vi "svx_Matched Index.vi"(11 "channel property":T1[](array[typedef]) {"probe angle [deg]" max=360; "direction" items=["CCW", "CW"]}) -> (0 "single index":i32[](array[numeric]), 1 "single list":u32[](array[numeric]), 2 "pair index":cluster{"index 1":i32, "index 2":i32}[](array[cluster]), 3 "new pair list":u32[](array[numeric]), 4 "direction error":bool, 6 "pair error":bool)   [LabVIEW 2017]
uses:
  <vilib>/addons/Sound and Vibration/Order Analysis/Data Presentation/SubVIs/OAT MCM Channel Property.ctl
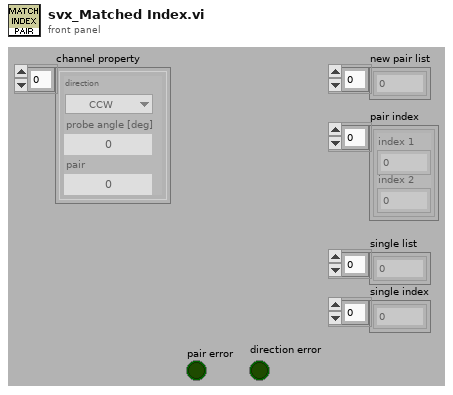
[diagram p1: front panel]
types:
  T1 = typedef "OAT MCM Channel Property.ctl" = cluster{"direction":u16, "probe angle [deg]":u16, "pair":u16}
  T2 = cluster{"index of element":i32, "index of element":i32}[]
  T3 = cluster{"index of element":i32, "index of element":i32}
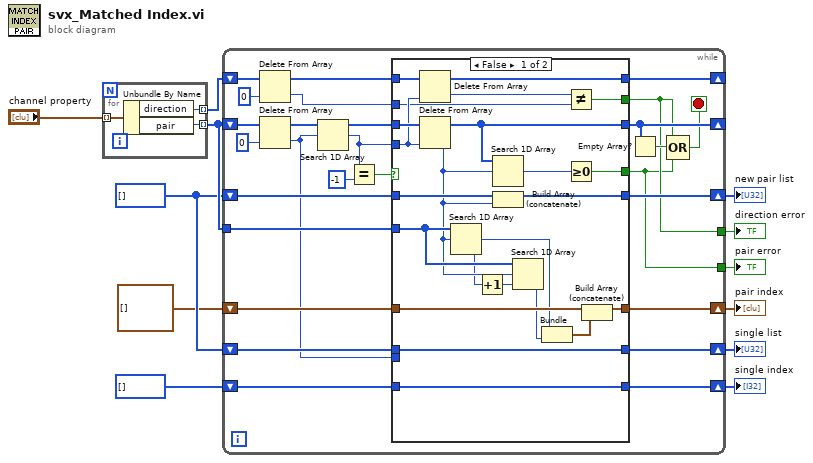
[diagram p0: block diagram]
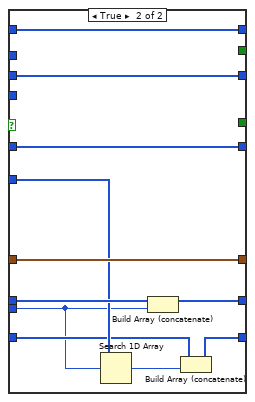
[diagram p2: hidden frame]
diagram:
  w9 = u32[] []
  n1 = for {
    tunnel: "channel property" -> [w15] mode=indexing
    tunnel: [w14] -> w10 mode=indexing
    tunnel: [w13] -> w3 mode=indexing
    n2 = Unbundle By Name(w15) -> ("direction"=w13:u16, "pair"=w14:u16)
  }
  n3 = while {
    shift-right: [w35] -> _
    shift-left: w10 -> [w34]
    shift-right: [w37] -> w11
    shift-left: w9 -> [w36]
    shift-right: [w33] -> w4
    shift-left: T2 [] -> [w32]
    tunnel: w10 -> [w31]
    shift-right: [w29] -> w6
    shift-left: w9 -> [w30]
    shift-right: [w26] -> w7
    shift-left: i32[] [] -> [w27]
    shift-right: [w19] -> _
    shift-left: w3 -> [w21]
    tunnel: [w17] -> w2
    tunnel: [w16] -> w1
    stop <- w23 stop-if-true
    n4 = Delete From Array(array=w21, index=0) -> (deleted portion=w18:u16, array with subset deleted=w20:u16[])  [unwired: 1 in]
    n5 = Delete From Array(array=w34, index=0) -> (deleted portion=w28:u16, array with subset deleted=w38:u16[])  [unwired: 1 in]
    n6 = Search 1D Array(1D array=w38, element=w28) -> (index of element=w25:i32)  [unwired: 1 in]
    n7 = Equal?(x=w25, y=-1) -> (x = y?=w39:bool)
    n8 = case shown="False" w39 {
      tunnel: [w54 w74] -> w35
      tunnel: w38 -> [w63 w74]
      tunnel: [w62 w73] -> w37
      tunnel: w36 -> [w61 w73]
      tunnel: w31 -> [w59 w69]
      tunnel: w32 -> [w58 w72]
      tunnel: [w57 w72] -> w33
      tunnel: w30 -> [w56 w71]
      tunnel: [w56 w70] -> w29
      tunnel: w28 -> [_ w65]
      tunnel: w27 -> [w55 w67]
      tunnel: [w55 w66] -> w26
      tunnel: w25 -> [w47 _]
      tunnel: [w51 _] -> w16
      tunnel: w20 -> [w46 w64]
      tunnel: [w45 w64] -> w19
      tunnel: w18 -> [w43 _]
      tunnel: [w42 _] -> w17
      frame False {
        n9 = Delete From Array(array=w46, index=w47) -> (deleted portion=w44:u16, array with subset deleted=w45:u16[])  [unwired: 1 in]
        n10 = Delete From Array(array=w63, index=w47) -> (deleted portion=w53:u16, array with subset deleted=w54:u16[])  [unwired: 1 in]
        n11 = Search 1D Array(1D array=w59, element=w53) -> (index of element=w50:i32)  [unwired: 1 in]
        n12 = Increment(x=w50) -> (x+1=w60:i32)
        n13 = Search 1D Array(1D array=w54, element=w53) -> (index of element=w52:i32)  [unwired: 1 in]
        n14 = Build Array (concatenate)(w61, w53) -> (w62:u32[])
        n15 = Search 1D Array(1D array=w59, element=w53, start index (0)=w60) -> (index of element=w49:i32)
        n16 = Bundle("index of element"=w50, "index of element"=w49) -> (w48:T3)  [unwired: 1 in]
        n17 = Not Equal?(x=w44, y=w43) -> (x != y?=w42:bool)
        n18 = Greater Or Equal To 0?(x=w52) -> (x >= 0?=w51:bool)
        n19 = Build Array (concatenate)(w58, w48) -> (w57:T2)
      }
      frame True {
        n20 = Search 1D Array(1D array=w69, element=w65) -> (index of element=w68:i32)  [unwired: 1 in]
        n21 = Build Array (concatenate)(w71, w65) -> (w70:u32[])
        n22 = Build Array (concatenate)(w67, w68) -> (w66:i32[])
      }
    }
    n23 = Empty Array?(array=w35) -> (empty?=w24:bool)
    n24 = Compound Arithmetic op=OR(w17, w24, w16) -> (w23:bool)
  }
  "new pair list" <- w11
  "single list" <- w6
  "single index" <- w7
  "direction error" <- w2
  "pair index" <- w4
  "pair error" <- w1
